vi "ParseContents.vi"(5 "body":string, 6 "error in":errorcluster) -> (0 "error out":errorcluster, 4 "contents":T1[](array[typedef]))   [LabVIEW 2014, in "Raspberry Pi Compatible Compiler for LabVIEW.lvlib" / "GitHub API.lvlib"]
uses:
  GitHub API.lvlib
  TypeDefs/GitHubContents_TD.ctl
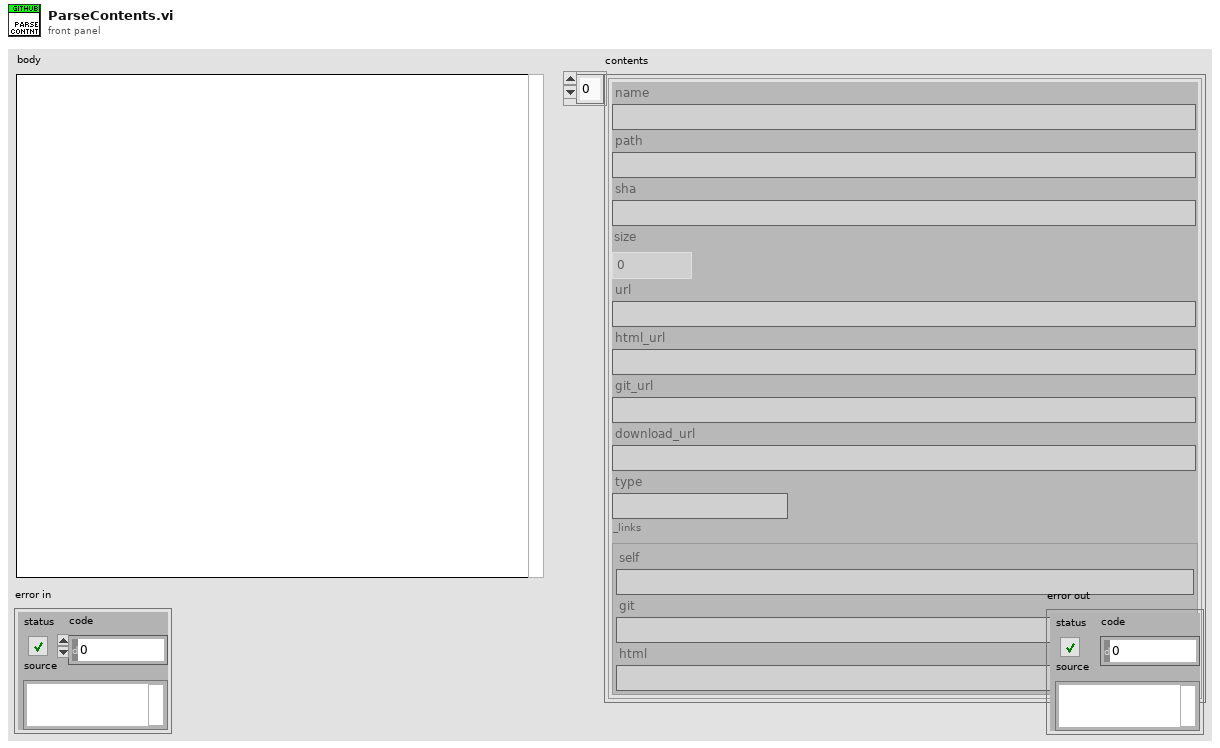
[diagram p1: front panel]
types:
  T1 = typedef "Raspberry Pi Compatible Compiler for LabVIEW.lvlib/GitHub API.lvlib/GitHubContents_TD.ctl" = cluster{"name":string, "path":string, "sha":string, "size":dbl, "url":string, "html_url":string, "git_url":string, "download_url":string, "type":string, "_links":cluster{"self":string, "git":string, "html":string}}
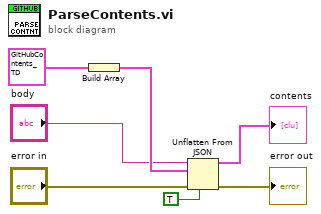
[diagram p0: block diagram]
diagram:
  n1 = Build Array(T1 {"name"="", "path"="", "sha"="", "size"=0.0, "url"="", "html_url"="", "git_url"="", "download_url"="", "type"="", "_links"={"self"="", "git"="", "html"=""}}) -> (w6:T1[])
  n2 = Unflatten From JSON(JSON string="body", type and defaults=w6, default null elements? (F)=TRUE, error in (no error)="error in") -> (value=→"contents":T1[], error out=→"error out":errorcluster)  [unwired: 3 in]
